vi "Get SLSC Switch Properties (SET 2010).vi"(8 "error in (no error)":errorcluster, 10 "Base Channels":i32=4, 11 "device":refnum<k21>="SLSC-12001-0317E1AA-Mod2") -> (0 "error out":errorcluster, 2 "SET Chxn Properties":cluster{"name":string, "value":i32}[](array[cluster]), 3 "SET Chxp Properties":cluster{"name":string, "value":i32}[](array[cluster]))   [LabVIEW 2019, in "SLSC Switch System Tests.lvclass"]
uses:
  SLSC Switch System Tests.lvclass
  <vilib>/SLSC/Initialize Session with Devices.vi
  <vilib>/SLSC/Get Phys Chan Property (Bool).vi
  <vilib>/SLSC/Close Session.vi
  <vilib>/SLSC/SLSC.lvlib
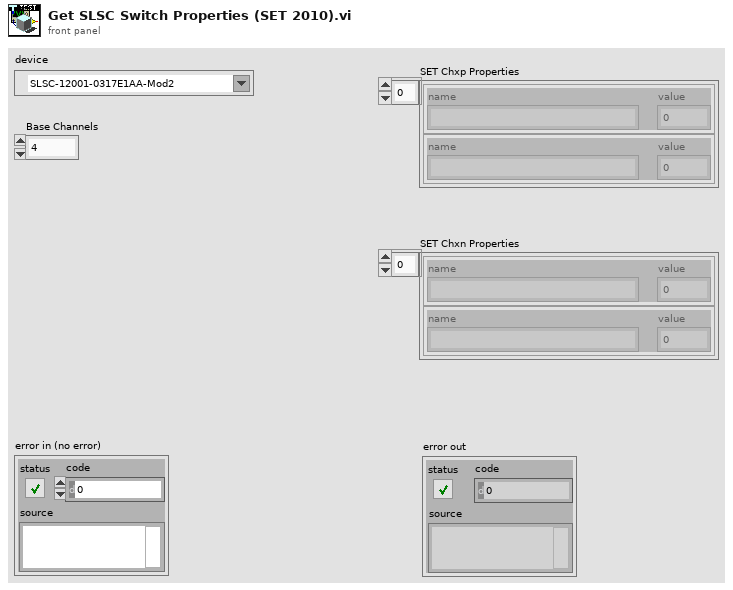
[diagram p1: front panel]
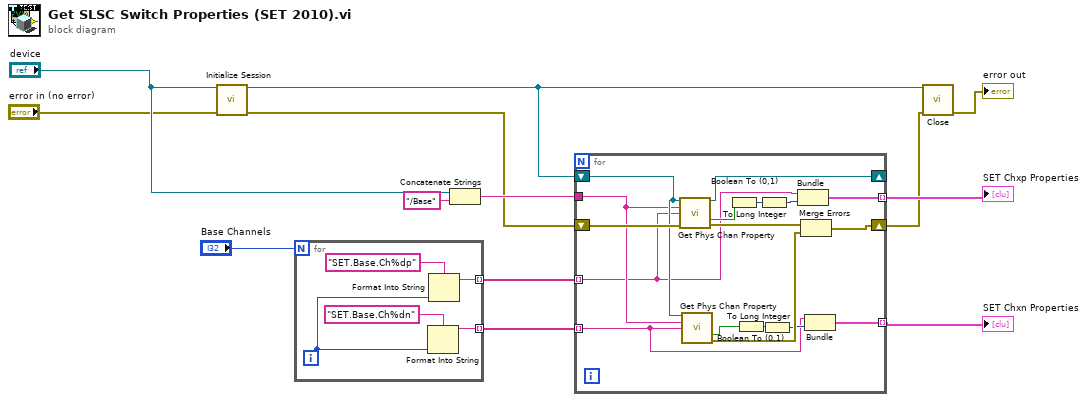
[diagram p0: block diagram]
diagram:
  n1 = call-poly <vilib>:"Initialize Session.vi"("devices"="device", "error in (no error)"="error in (no error)") -> ("session out"=w9:refnum<k21>, "error out"=w7:errorcluster)  [unwired: 12 in]
  n2 = for {
    N: "Base Channels" -> [_]
    tunnel: [w15] -> w6 mode=indexing
    tunnel: [w14] -> w5 mode=indexing
    i -> [w16]
    n3 = Format Into String(format string="SET.Base.Ch%dn" ("string"), w16) -> (resulting string=w15:string)  [unwired: 2 in, 1 out]
    n4 = Format Into String(format string="SET.Base.Ch%dp" ("string"), w16) -> (resulting string=w14:string)  [unwired: 2 in, 1 out]
  }
  n5 = Concatenate Strings("device", "/Base" ("string")) -> (w8:string)
  n6 = for {
    tunnel: w8 -> [w33]
    shift-right: [w30] -> w2
    shift-left: w7 -> [w35]
    tunnel: w6 -> [w23] mode=indexing
    tunnel: w5 -> [w22] mode=indexing
    shift-right: [w21] -> _
    shift-left: w9 -> [w34]
    tunnel: [w20] -> w4 mode=indexing
    tunnel: [w19] -> w3 mode=indexing
    n7 = call-poly <vilib>:"Get Phys Chan Property.vi"("session in"=w34, "physical channels"=w33, "property"=w22, "error in (no error)"=w35) -> ("session out"=w21:refnum<k21>, "property value"=w28:bool, "error out"=w32:errorcluster)  [unwired: 9 in]
    n8 = call-poly <vilib>:"Get Phys Chan Property.vi"("session in"=w34, "physical channels"=w33, "property"=w23) -> ("property value"=w27:bool, "error out"=w31:errorcluster)  [unwired: 10 in, 1 out]
    n9 = Boolean To (0,1)(Boolean=w28) -> (0, 1=w29:i16)
    n10 = Boolean To (0,1)(Boolean=w27) -> (0, 1=w25:i16)
    n11 = To Long Integer(number=w29) -> (32bit integer=w26:i32)
    n12 = To Long Integer(number=w25) -> (32bit integer=w24:i32)
    n13 = Bundle(w22, w26) -> (w20:cluster{string, i32})  [unwired: 1 in]
    n14 = Merge Errors(w32, w31) -> (w30:errorcluster)
    n15 = Bundle(w23, w24) -> (w19:cluster{string, i32})  [unwired: 1 in]
  }
  "SET Chxp Properties" <- w4
  "SET Chxn Properties" <- w3
  n16 = call-poly <vilib>:"Close.vi"("session in"=w9, "error in (no error)"=w2) -> ("error out"=→"error out":errorcluster)  [unwired: 13 in]
